vi "FisherPaykel Spin Setup.vi"(8 "Error In":errorcluster, 10 "Motor Profile Data":T1, 11 "Spin Profile in":T2 {"Running Time (s)" step=1; "Acceleration Rate - (10 Slowest/1000 Fastest)" min=10 max=1000 step=1; "Target Speed (RPM)" min=23 max=1600 step=1}) -> (0 "Error Out":errorcluster, 1 "Spin Profile out":T2 {"Running Time (s)" step=1; "Acceleration Rate - (10 Slowest/1000 Fastest)" min=10 max=1000 step=1; "Target Speed (RPM)" min=23 max=1600 step=1}, 3 "States Out":string)   [LabVIEW 2016]
uses:
  Type Definitions/Fisher Paykel Motor Profile.ctl
  Type Definitions/FisherPaykel Direction CMD.ctl
  Type Definitions/FisherPaykel Motor Profile Data ERD.ctl
panel:
  # "Spin Profile Parameters"
  # "Spin Start Parameters"
  # "Spin Profile Parameters"
  # "Spin Start Parameters"
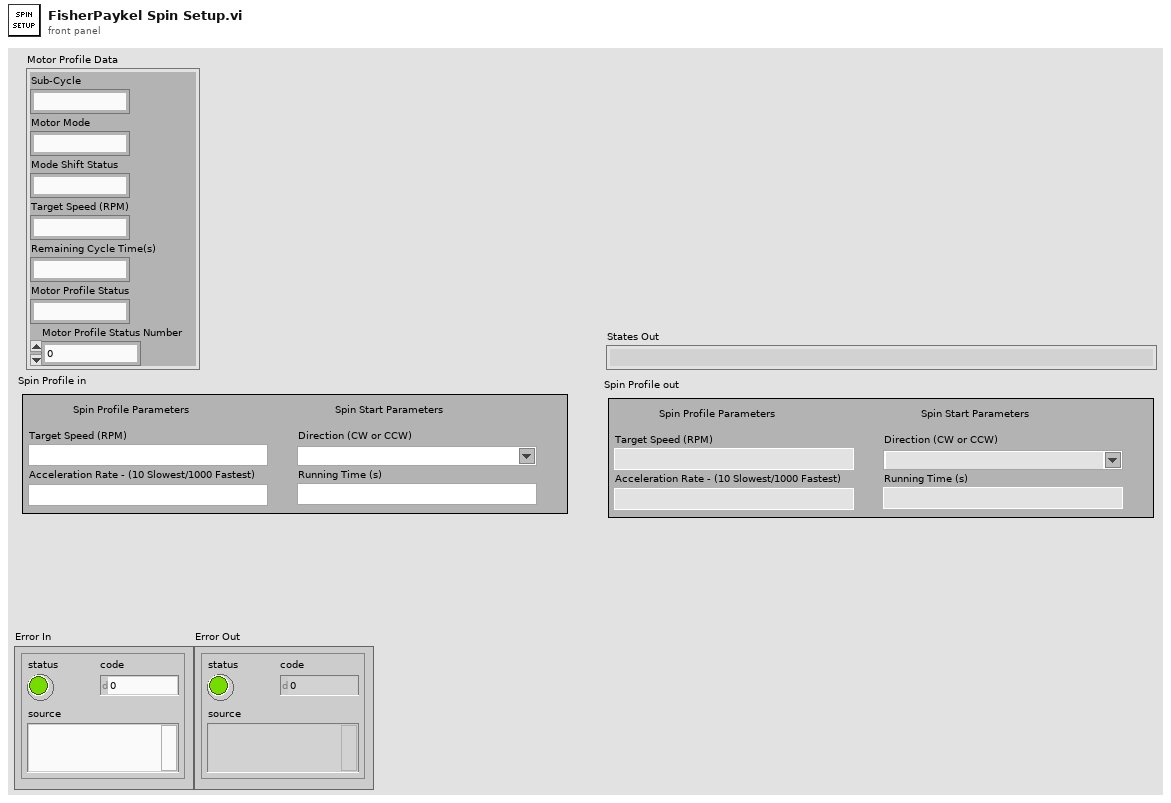
[diagram p1: front panel]
types:
  T1 = typedef "FisherPaykel Motor Profile Data ERD.ctl" = cluster{"Sub-Cycle":string, "Motor Mode":string, "Mode Shift Status":string, "Target Speed (RPM)":string, "Remaining Cycle Time(s)":string, "Motor Profile Status":string, "Motor Profile Status Number":u16}
  T2 = typedef "Fisher Paykel Motor Profile.ctl" = cluster{"Target Speed (RPM)":u16, "Acceleration Rate - (10 Slowest/1000 Fastest)":u16, "Running Time (s)":u16, "Direction (CW or CCW)":T3}
  T3 = typedef "FisherPaykel Direction CMD.ctl" = string
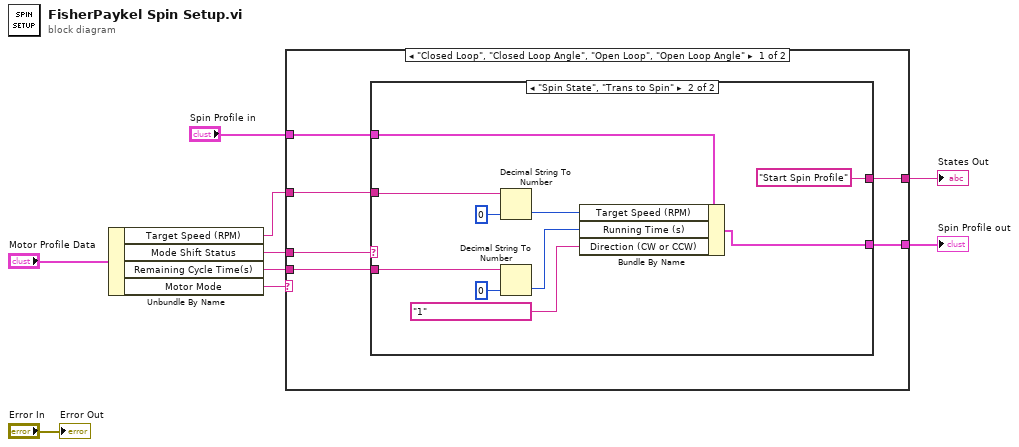
[diagram p0: block diagram]
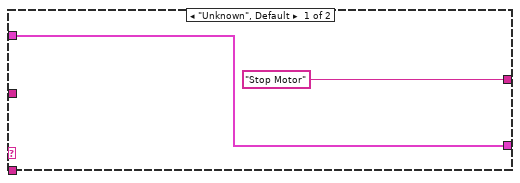
[diagram p2: hidden frame]
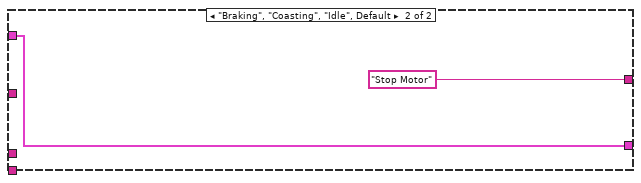
[diagram p3: hidden frame]
diagram:
  n1 = Unbundle By Name("Motor Profile Data") -> ("Target Speed (RPM)"=w1:string, "Mode Shift Status"=w4:string, "Remaining Cycle Time(s)"=w3:string, "Motor Mode"=w2:string)
  n2 = case shown="\"Closed Loop\", \"Closed Loop Angle\", \"Open Loop\", \"Open Loop Angle\"" w2 {
    tunnel: [w12 "Stop Motor"] -> w7
    tunnel: "Spin Profile in" -> [w15 w28]
    tunnel: [w14 w28] -> w9
    tunnel: w4 -> [w13 _]
    tunnel: w1 -> [w11 _]
    tunnel: w3 -> [w10 _]
    frame "Closed Loop", "Closed Loop Angle", "Open Loop", "Open Loop Angle" {
      n3 = case shown="\"Spin State\", \"Trans to Spin\"" w13 {
        tunnel: w15 -> [w17 w27]
        tunnel: [w17 w26] -> w14
        tunnel: ["Stop Motor" "Start Spin Profile"] -> w12
        tunnel: w11 -> [_ w21]
        tunnel: w10 -> [_ w19]
        frame "Unknown", Default {
        }
        frame "Spin State", "Trans to Spin" {
          n4 = Decimal String To Number(string=w21, default (0L)=u16 0 ("default (0 I32)")) -> (number=w22:u16)  [unwired: 1 in, 1 out]
          n5 = Decimal String To Number(string=w19, default (0L)=u16 0 ("default (0 I32)")) -> (number=w18:u16)  [unwired: 1 in, 1 out]
          n6 = Bundle By Name(cluster=w27, "Target Speed (RPM)"=w22, "Running Time (s)"=w18, "Direction (CW or CCW)"=T3 "1") -> (w26:T2)
        }
      }
    }
    frame "Braking", "Coasting", "Idle", Default {
    }
  }
  "Spin Profile out" <- w9
  "States Out" <- w7
  "Error Out" <- "Error In"
